vi "checkError.vi"(8 "error in (no error)":errorcluster, 10 "Equipo_Medicion in":T1={"ID_EQUIPO"=0, "IP_EQUIPO"="", "NOMBRE_EQUIPO"="", "ESTADO_EQUIPO"="", "DESCRIPCION"="", "ID_MEDICION"=0, "ESTADO_MEDICION"="", "TIEMPO_MEDICION"="12-02-2019 18:41"}) -> (0 "error out":errorcluster, 5 "ESTADO_EQUIPO":string)   [LabVIEW 2018]
uses:
  Controls/Equipos_Medicion_cluster.ctl
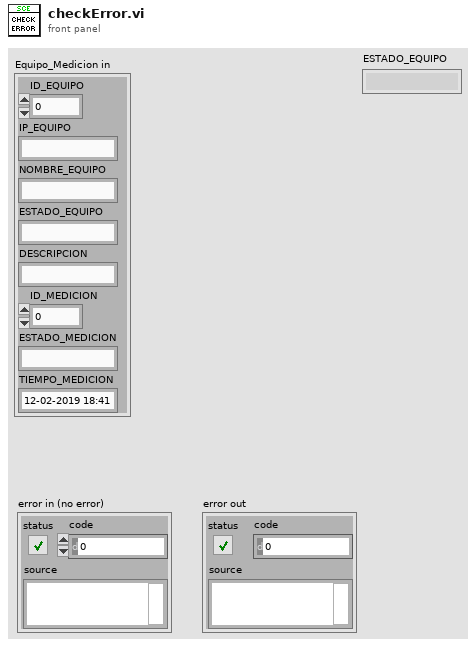
[diagram p1: front panel]
types:
  T1 = typedef "Equipos_Medicion_cluster.ctl" = cluster{"ID_EQUIPO":i32, "IP_EQUIPO":string, "NOMBRE_EQUIPO":string, "ESTADO_EQUIPO":string, "DESCRIPCION":string, "ID_MEDICION":i32, "ESTADO_MEDICION":string, "TIEMPO_MEDICION":string}
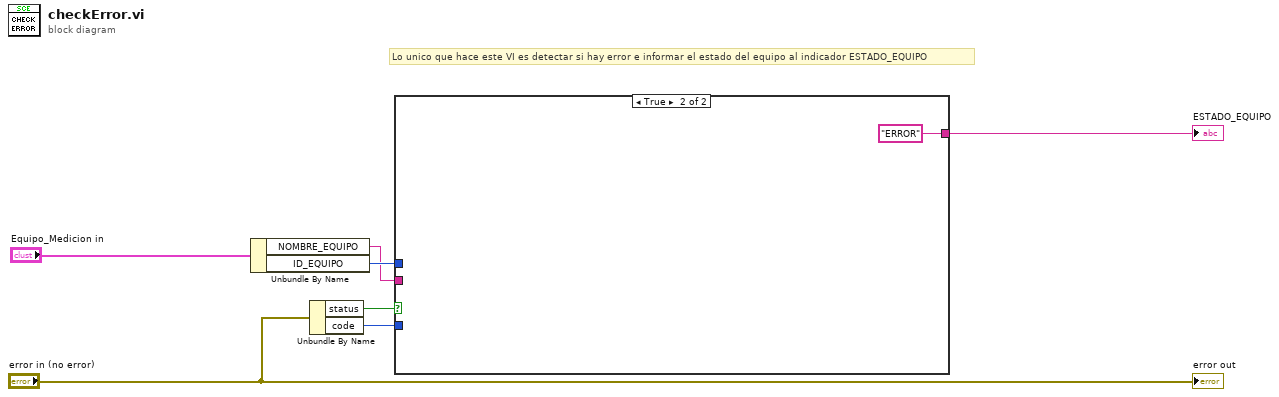
[diagram p0: block diagram]
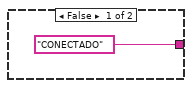
[diagram p2: hidden frame]
diagram:
  # "Lo unico que hace este VI es detectar si hay error e informar el estado del equipo al indicador ESTADO_EQUIPO"
  n1 = Unbundle By Name("Equipo_Medicion in") -> ("NOMBRE_EQUIPO"=w2:string, "ID_EQUIPO"=w3:i32)
  n2 = Unbundle By Name("error in (no error)") -> ("status"=w6:bool, "code"=w5:i32)
  n3 = case shown="True" w6 {
    tunnel: w5 -> [_ _]
    tunnel: ["CONECTADO" "ERROR"] -> w1
    tunnel: w3 -> [_ _]
    tunnel: w2 -> [_ _]
    frame False {
    }
    frame True {
    }
  }
  "ESTADO_EQUIPO" <- w1
  "error out" <- "error in (no error)"
